vi "_CSMObj-Obtain Chain.vi"(8 "error in (no error)":errorcluster, 11 "Requested Name":string) -> (0 "error out":errorcluster, 3 "CSMQ Out":T1)   [LabVIEW 2017, in "Communicable State Machine.lvlib"]
uses:
  Communicable State Machine.lvlib
  _CSMObj.ctl
  _CSMObj-Info.ctl
  Typedef/_CSM_MODE.ctl
  _CSMObj-Refs.ctl
  _CSMObj-Data.ctl
  Priority Queue/Priority Queue.ctl
  Typedef/_Cross CSM State Data.ctl
  Typedef/_CSM_MSG_TYPE.ctl
  Typedef/_Cross CSM State Response.ctl
  Typedef/_CSM_Response Source Message.ctl
  Priority Queue/def-Data(LowPRI-Q).ctl
  _CSMObj-ModeData.ctl
  Typedef/_CSM Status Change Event Data.ctl
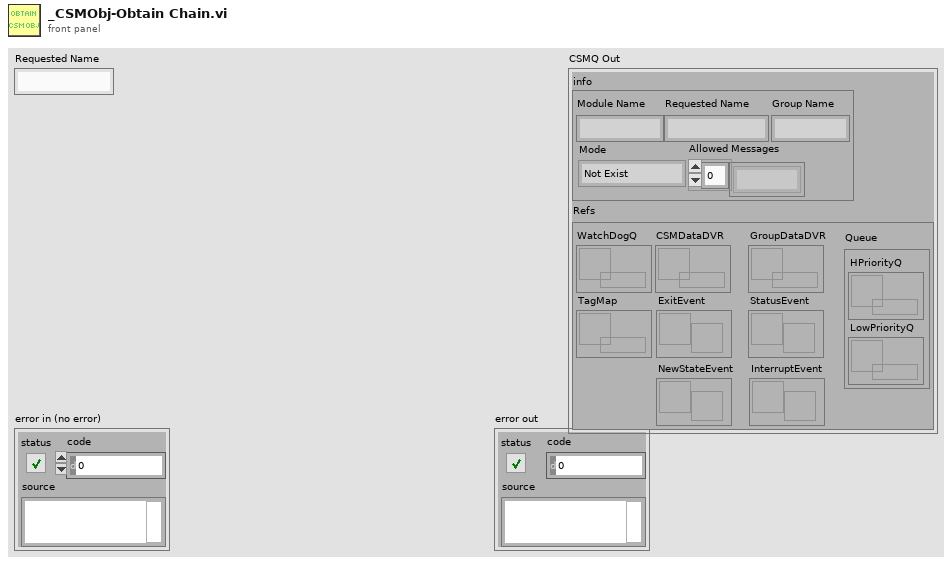
[diagram p1: front panel]
types:
  T1 = typedef "Communicable State Machine.lvlib/_CSMObj.ctl" = cluster{"info":T2, "Refs":T4}
  T2 = typedef "Communicable State Machine.lvlib/_CSMObj-Info.ctl" = cluster{"Module Name":string, "Requested Name":string, "Group Name":string, "Mode":T3, "Allowed Messages":string[]}
  T3 = typedef "Communicable State Machine.lvlib/_CSM_MODE.ctl" = enum16{"Not Exist", "Stand Alone", "CSM", "Worker", "Worker Agent", "Chain Node", "Chain"}
  T4 = typedef "Communicable State Machine.lvlib/_CSMObj-Refs.ctl" = cluster{"WatchDogQ":refnum<queue>, "CSMDataDVR":refnum<data-value>, "Queue":T5, "GroupDataDVR":refnum<data-value>, "TagMap":refnum<data-value>, "ExitEvent":refnum<user-event>, "NewStateEvent":refnum<user-event>, "StatusEvent":refnum<user-event>, "InterruptEvent":refnum<user-event>}
  T5 = typedef "Communicable State Machine.lvlib/Priority Queue.ctl" = cluster{"HPriorityQ":refnum<queue>, "LowPriorityQ":refnum<queue>}
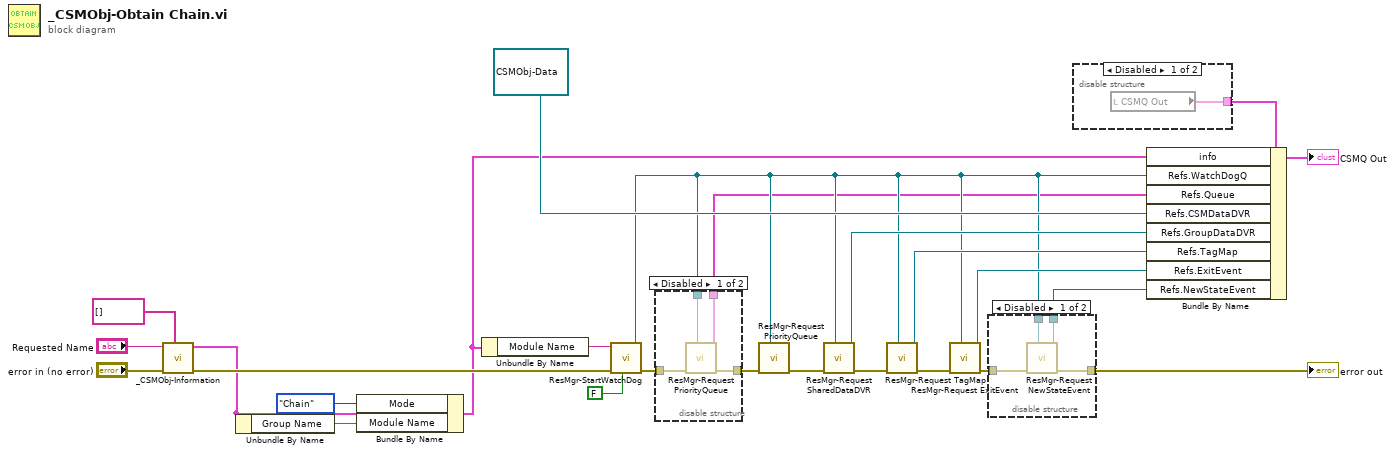
[diagram p0: block diagram]
diagram:
  n1 = call "_CSMObj-Information.vi"("Allowed Messages (Empty For All)"=string[] [] ("Allowed Messages(Empty for all)"), "Error In"="error in (no error)", "Requested Name"="Requested Name") -> ("error out"=w12:errorcluster, "CSMO-Info"=w3:T2)  [unwired: 7 in]
  n2 = Unbundle By Name(w3) -> ("Group Name"=w2:string)
  n3 = Bundle By Name(cluster=w3, "Mode"=_CSM_MODE."Chain", "Module Name"=w2) -> (w5:T2)
  n4 = Unbundle By Name(w5) -> ("Module Name"=w20:string)
  n5 = call "ResMgr-StartWatchDog.vi"("Force?"=FALSE, "error in (no error)"=w12, "ModuleName"=w20) -> ("error out"=w13:errorcluster, "WatchDogQ"=w7:refnum<queue>)  [unwired: 7 in]
  n6 = disable-structure shown="Disabled" {
    disable-tunnel: w13 -> [w30 w31]
    disable-tunnel: [w29 w31] -> w8
    disable-tunnel: w7 -> [w28 _]
    disable-tunnel: [w27 _] -> w6
    frame Disabled {
      n7 = call "ResMgr-Request PriorityQueue.vi"("WatchDogQ"=w28, "Error In"=w30) -> ("error out"=w29:errorcluster, "Priority Queue"=w27:T5)  [unwired: 8 in]
    }
    frame Enabled {
    }
  }
  n8 = call "ResMgr-Request PriorityQueue.vi"("WatchDogQ"=w7, "Error In"=w8) -> ("error out"=w10:errorcluster)  [unwired: 8 in, 1 out]
  n9 = call "ResMgr-Request SharedDataDVR.vi"("WatchDogQ"=w7, "Error In"=w10) -> ("error out"=w17:errorcluster, "DVR"=w18:refnum<data-value>)  [unwired: 8 in]
  n10 = call "ResMgr-Request TagMap.vi"("WatchDogQ"=w7, "Error In"=w17) -> ("error out"=w15:errorcluster, "Data Value Reference"=w21:refnum<data-value>)  [unwired: 8 in]
  n11 = call "ResMgr-Request ExitEvent.vi"("WatchDogQ"=w7, "Error In"=w15) -> ("error out"=w14:errorcluster, "CSMExit"=w22:refnum<user-event>)  [unwired: 8 in]
  n12 = disable-structure shown="Disabled" {
    disable-tunnel: [w35 _] -> w16
    disable-tunnel: w14 -> [w34 w36]
    disable-tunnel: [w33 w36] -> w11
    disable-tunnel: w7 -> [w32 _]
    frame Disabled {
      n13 = call "ResMgr-Request NewStateEvent.vi"("WatchDogQ"=w32, "Error In"=w34) -> ("error out"=w33:errorcluster, "User Event Out"=w35:refnum<user-event>)  [unwired: 8 in]
    }
    frame Enabled {
    }
  }
  "error out" <- w11
  n14 = disable-structure shown="Disabled" {
    disable-tunnel: [w37 _] -> w19
    frame Disabled {
      n15 = local read "CSMQ Out"() -> (w37:T1)
    }
    frame Enabled {
    }
  }
  n16 = Bundle By Name(cluster=w19, "info"=w5, "Refs.WatchDogQ"=w7, "Refs.Queue"=w6, "Refs.CSMDataDVR"=refnum<data-value> refnum ("Refs.CSM-Data"), "Refs.GroupDataDVR"=w18, "Refs.TagMap"=w21, "Refs.ExitEvent"=w22, "Refs.NewStateEvent"=w16) -> (→"CSMQ Out":T1)
